vi "Multistation Example.vi"() -> ()   [LabVIEW 2019]
uses:
  Test Bench Tools.lvlib
panel:
  in  "Launch Test 2":bool
  out "Result_Station2":T1(array[cluster])
  out "Result_Station1":T1(array[cluster])
  in  "Launch Test":bool
  in  "Stop":bool
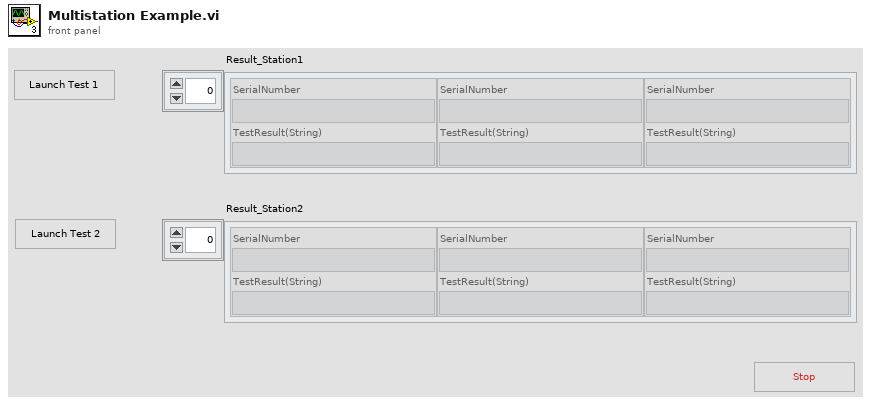
[diagram p1: front panel]
types:
  T1 = cluster{"SerialNumber":string, "TestResult(String)":string}[]
  T2 = enum16{"Station 1", "Station 2", "Station 3", "Station 4"}
  T3 = cluster{"new reference":refnum<k24>, "Array":refnum<k27>[], "Mgessage":refnum<user-event>}
  T4 = enum32{"Invalid", "Standard", "Closed", "Hidden", "Minimized", "Maximized"}
  T5 = enum32{"invalid app kind", "Development System", "Run Time System", "Student Edition", "Embedded LabVIEW", "Evaluation", "Custom"}
  T6 = cluster{"Core":cluster{"Current VI Reference":refnum<vi>, "Close Panel on Exit?":bool}, "Your Boolean data":bool, "Your string data":string, "hWnd":u32}
  T7 = cluster{"Current VI Reference":refnum<vi>, "Close Panel on Exit?":bool}
  T8 = enum16{"None", "Top", "Bottom", "Left", "Right", "Left-Top", "Left-Bottom", "Right-Top", "Right-Bottom"}[]
  T9 = cluster{"SerialNumber":string, "TestResult(String)":string}
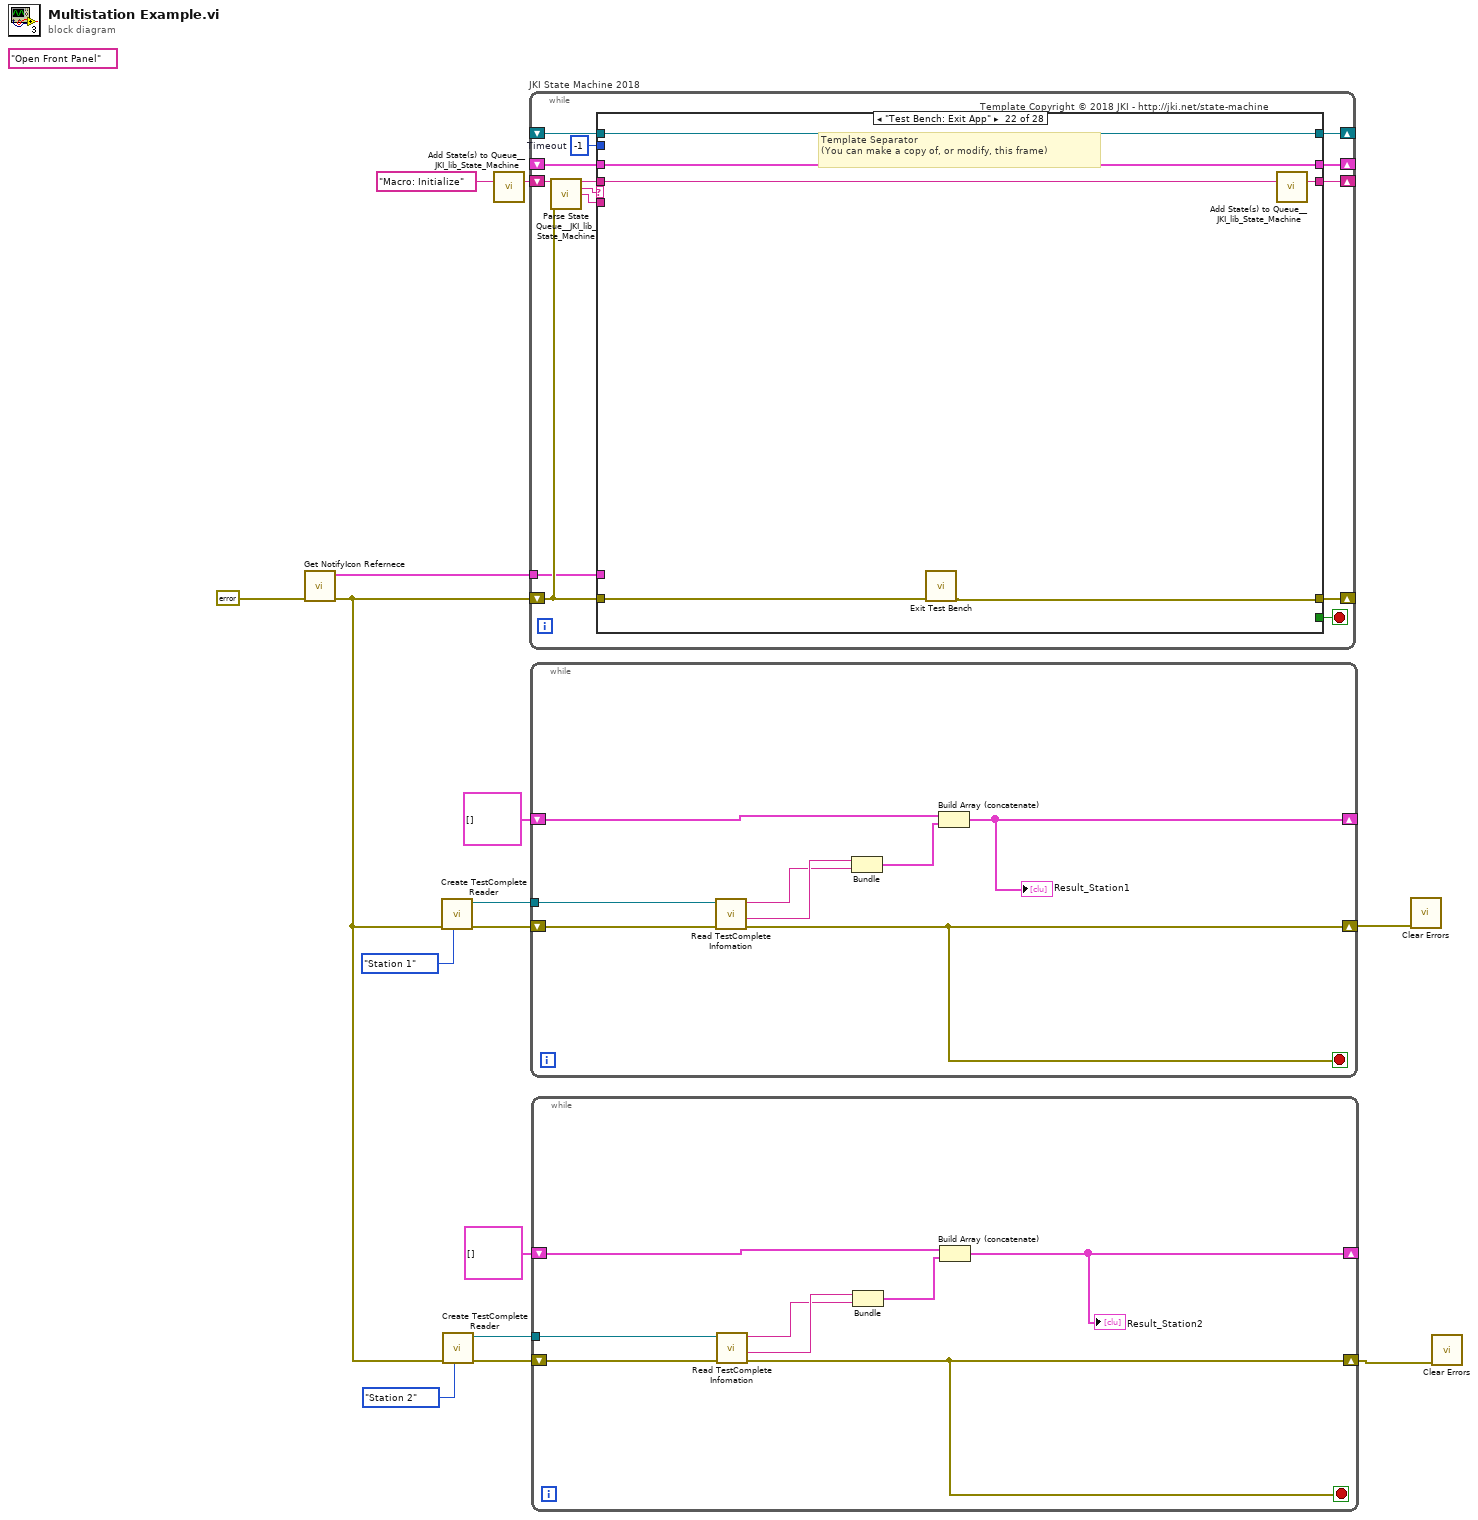
[diagram p0: block diagram]
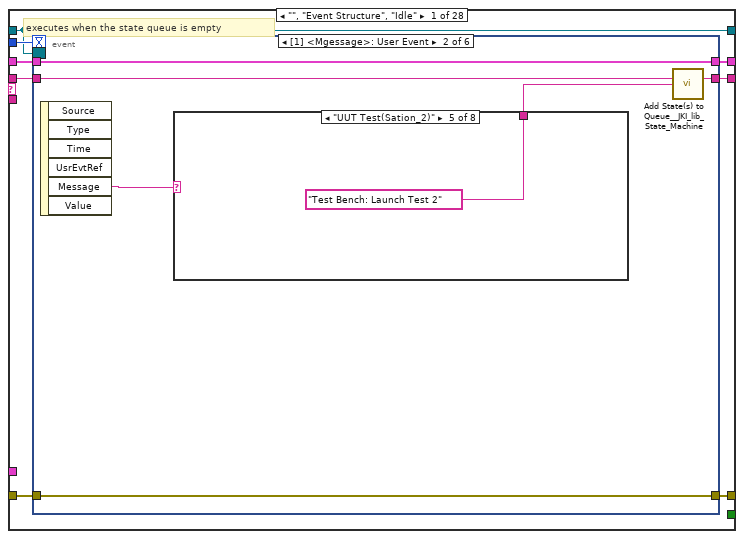
[diagram p2: hidden frame]
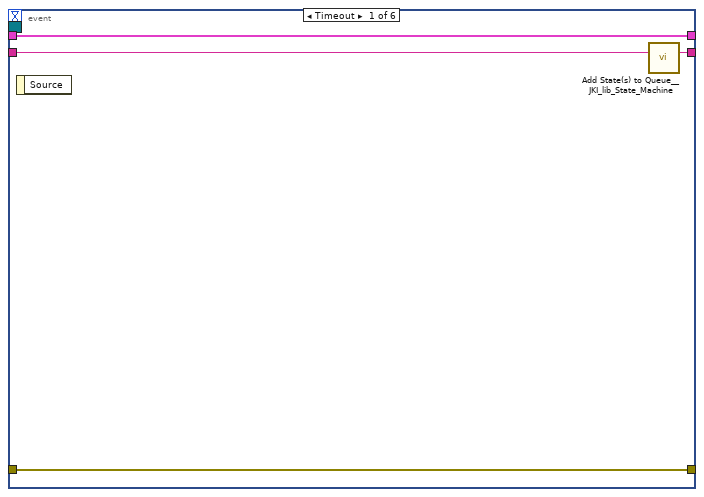
[diagram p3: hidden frame]
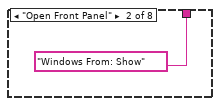
[diagram p5: hidden frame]
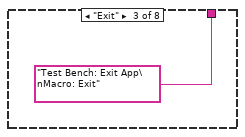
[diagram p6: hidden frame]
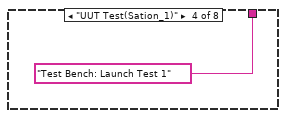
[diagram p7: hidden frame]
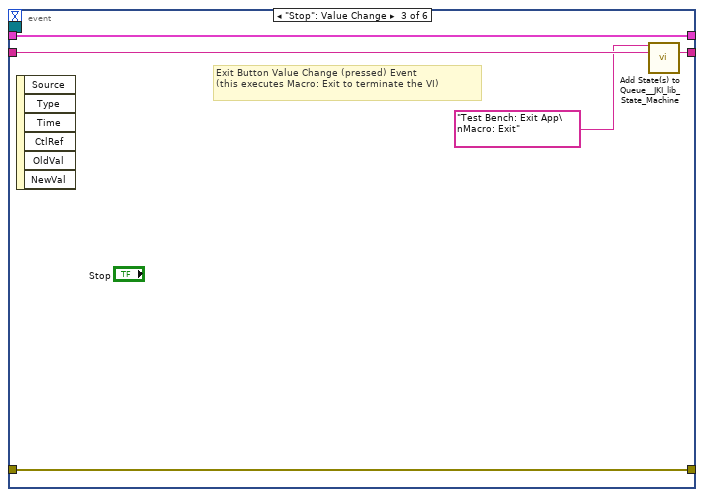
[diagram p11: hidden frame]
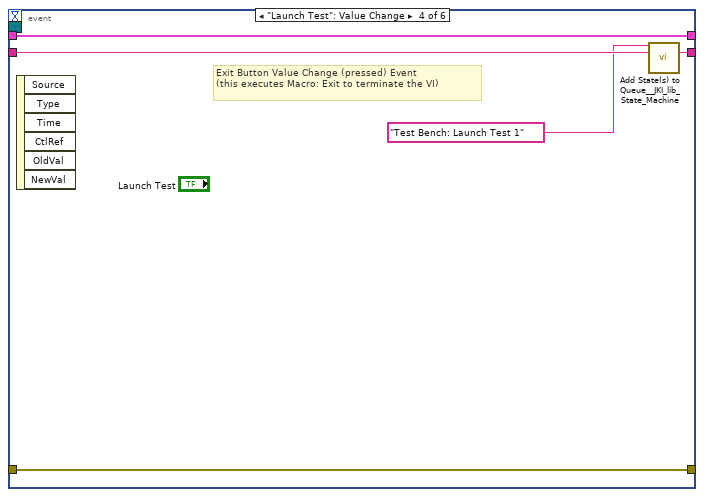
[diagram p12: hidden frame]
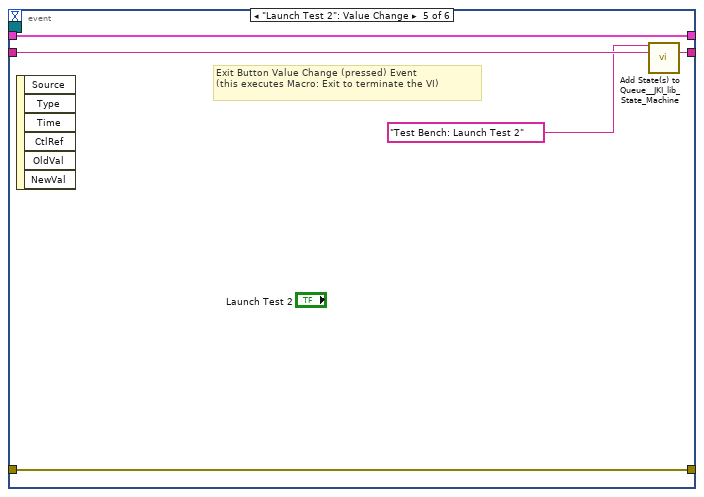
[diagram p13: hidden frame]
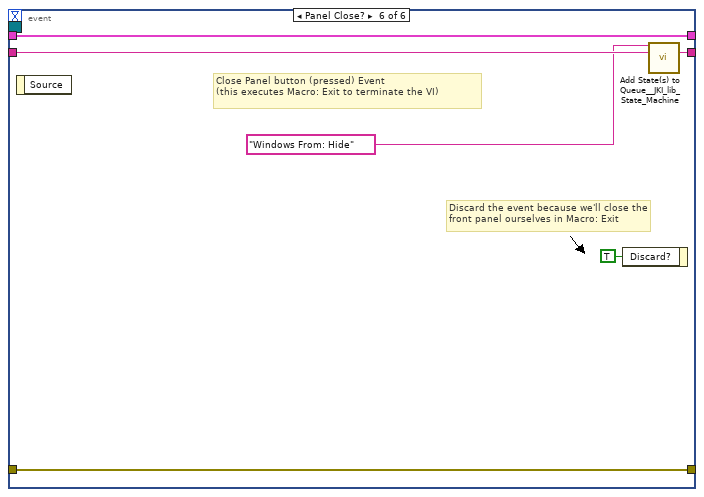
[diagram p14: hidden frame]
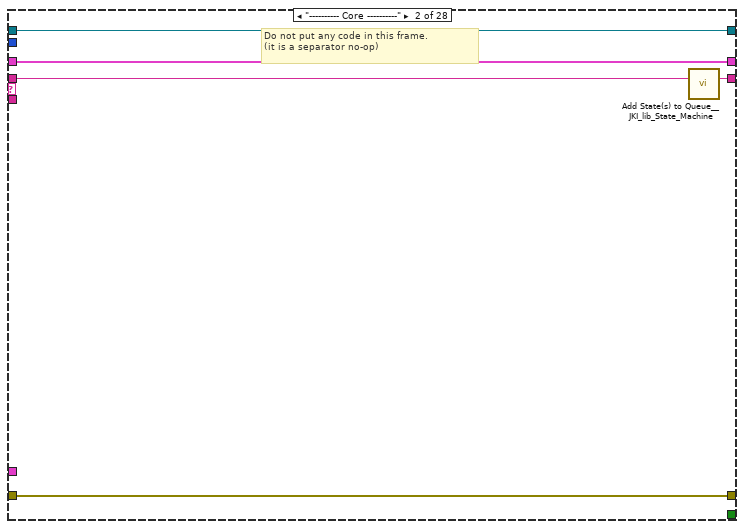
[diagram p15: hidden frame]
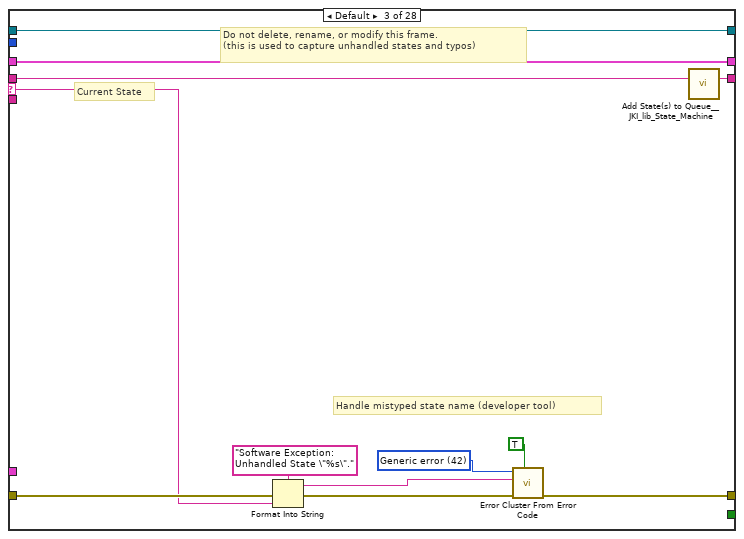
[diagram p16: hidden frame]
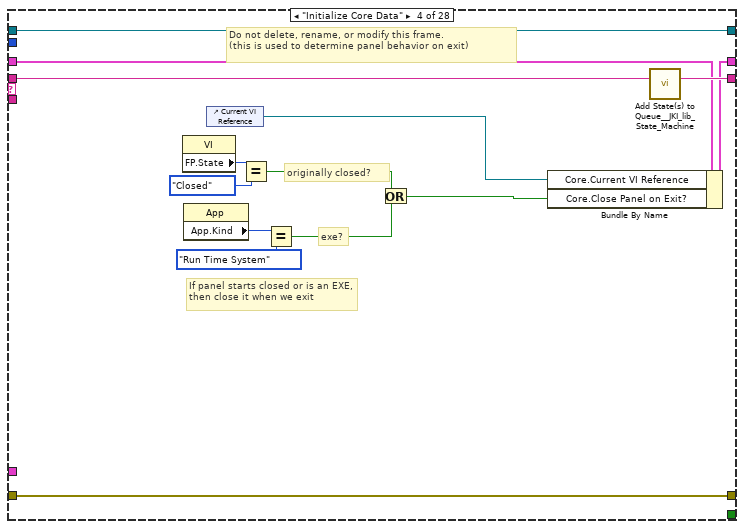
[diagram p17: hidden frame]
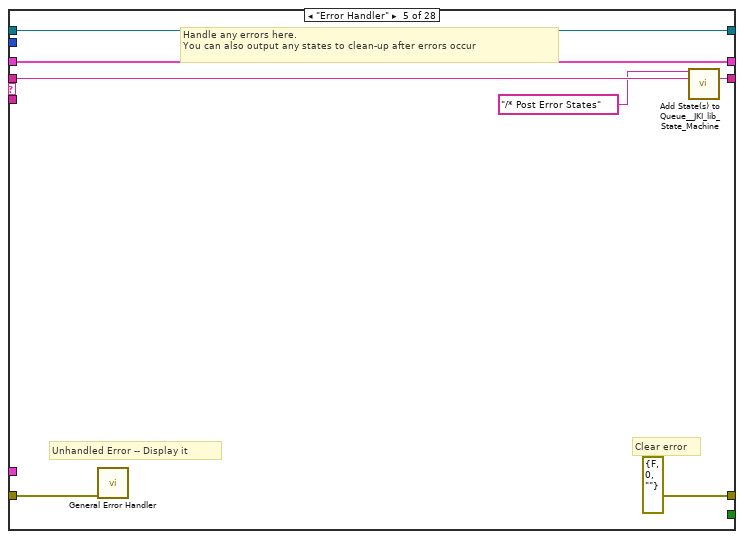
[diagram p18: hidden frame]
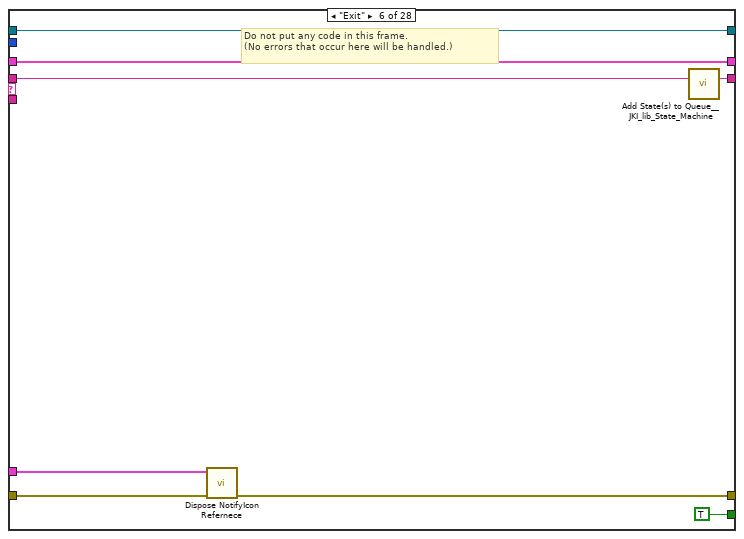
[diagram p19: hidden frame]
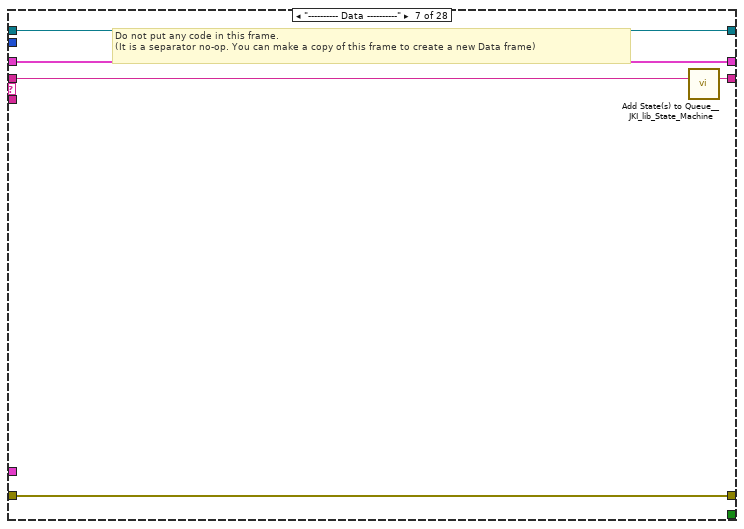
[diagram p20: hidden frame]
diagram:
  (unwired) "Open Front Panel" ("text")
  n1 = call "Get NotifyIcon Refernece.vi"("error in (no error)"=errorcluster {"status"=FALSE, "code"=0, "source"=""} ("error out")) -> ("error out"=w3:errorcluster, "reference out"=w9:T3)  [unwired: 9 in]
  n2 = call "Create TestComplete Reader.vi"("Station"=T2."Station 1", "error in (no error)"=w3) -> ("error out"=w13:errorcluster, "reader endpoint"=w11:refnum<k21>)  [unwired: 8 in]
  n3 = call "Create TestComplete Reader.vi"("Station"=T2."Station 2", "error in (no error)"=w3) -> ("error out"=w4:errorcluster, "reader endpoint"=w6:refnum<k21>)  [unwired: 8 in]
  n4 = call <vilib>:"Add State(s) to Queue__JKI_lib_State_Machine.vi"("State(s) in (\"\")"="Macro: Initialize") -> ("States Out"=w15:string)  [unwired: 14 in]
  n5 = while "JKI State Machine 2018" {
    shift-right: [w22] -> _
    shift-left: _ -> [w21]
    shift-right: [w25] -> _
    shift-left: w3 -> [w19]
    shift-right: [w24] -> _
    shift-left: w15 -> [w26]
    shift-right: [w18] -> _
    shift-left: _ -> [w17]
    tunnel: w9 -> [w16]
    stop <- w23 stop-if-true
    w20 = -1  # Timeout
    # "Template Copyright © 2018 JKI - http://jki.net/state-machine"
    n6 = call <vilib>:"Parse State Queue__JKI_lib_State_Machine.vi"("State Queue"=w26, "Error In (no error)"=w19) -> ("Remaining States"=w28:string, "Current State"=w29:string, "Arguments"=w27:string)  [unwired: 11 in]
    n7 = case shown="\"Test Bench: Exit App\"" w29 {
      selector: w29 -> [_ _ w79 _ _ _ _ _ _ _ _ _ _ _ _ _ _ _ _ _ _ _ _ _ _ _ _ _]
      tunnel: w28 -> [w37 w77 w83 w103 w110 w118 w123 w132 w139 w144 w152 w158 w163 w168 w175 w187 w257 w263 w274 w279 w286 w292 w300 w308 w313 w327 w344 w353]
      tunnel: w27 -> [_ _ _ _ _ _ _ _ _ _ _ _ _ _ w170 w181 _ _ _ _ _ _ _ _ _ _ _ _]
      tunnel: w21 -> [w35 w74 w81 w96 w107 w116 w120 _ w134 w141 w150 w156 w160 w166 w173 w183 w254 w260 w271 w276 w284 w290 w298 w306 w310 w323 w341 w347]
      tunnel: [w34 w75 w85 w100 errorcluster {"status"=FALSE, "code"=0, "source"=""} ("error out") w111 w121 w129 w135 w142 w148 w153 w161 w165 w171 w184 w255 w261 w272 w277 w282 w287 w293 w302 w309 w319 w329 w349] -> w25
      tunnel: w19 -> [w33 w75 w84 w100 w106 w112 w121 w129 w136 w142 w147 w154 w161 w165 w172 w185 w255 w261 w272 w277 w283 w289 w295 w303 w309 w324 w335 w350]
      tunnel: [w36 w76 w82 w102 w109 w117 w122 w131 w138 w143 w151 w157 w162 w167 w174 w186 w256 w262 w273 w278 w285 w291 w299 w307 w312 w326 w343 w352] -> w24
      tunnel: [_ _ _ _ _ TRUE _ _ _ _ _ _ _ _ _ _ _ _ _ _ _ _ _ _ _ _ _ _] -> w23
      tunnel: [w32 w74 w81 w101 w107 w116 w120 w130 w134 w141 w150 w156 w160 w166 w173 w183 w254 w260 w271 w276 w284 w290 w298 w306 w310 w323 w341 w345] -> w22
      tunnel: w20 -> [w31 _ _ _ _ _ _ _ _ _ _ _ _ _ _ _ _ _ _ _ _ _ _ _ _ _ _ _]
      tunnel: [w30 w73 w78 w90 w104 w114 w119 w125 w133 w140 w149 w155 w159 w164 w169 w180 w253 w258 w264 w275 w281 w288 w296 w304 w311 w325 w342 w351] -> w18
      tunnel: w17 -> [w30 w73 w78 w90 w104 w114 w119 w125 w133 w140 _ w155 w159 w164 w169 w180 w253 w258 w264 w275 w281 w288 w296 w304 w311 w325 w342 w351]
      tunnel: w16 -> [_ _ _ _ _ w113 _ _ _ _ w146 _ _ _ _ _ _ _ _ _ _ _ _ _ _ _ _ _]
      frame "", "Event Structure", "Idle" {
        # "executes when the state queue is empty"
        n8 = event shown="[1] <Mgessage>: User Event" {
          selector: w30 -> [_ _ _ _ _ _]
          dyn-events: _ -> [_ _ _ _ _ _]
          timeout: w31 -> [_ _ _ _ _ _]
          tunnel: w37 -> [w41 w47 w56 w61 w66 w72]
          tunnel: [w40 w46 w55 w60 w65 w71] -> w36
          tunnel: w35 -> [w38 w44 w53 w58 w63 w69]
          tunnel: [w39 w45 w54 w59 w64 w70] -> w34
          tunnel: w33 -> [w39 w45 w54 w59 w64 w70]
          tunnel: [w38 w44 w53 w58 w63 w69] -> w32
          event Timeout {
            n9 = event-data() -> ()  [unwired: 1 in, 1 out]
            n10 = call <vilib>:"Add State(s) to Queue__JKI_lib_State_Machine.vi"("State(s) in (\"\")"=w41) -> ("States Out"=w40:string)  [unwired: 14 in]
          }
          event User Event {
            n11 = event-data() -> ("Message"=w43:string)  [unwired: 1 in, 5 out]
            n12 = case shown="\"UUT Test(Sation_2)\"" w43 {
              tunnel: [_ "Windows From: Show" "Test Bench: Exit App\nMacro: Exit" "Test Bench: Launch Test 1" "Test Bench: Launch Test 2" _ _ _] -> w42
              frame "Idle", Default {
              }
              frame "Open Front Panel" {
              }
              frame "Exit" {
              }
              frame "UUT Test(Sation_1)" {
              }
              frame "UUT Test(Sation_2)" {
              }
              frame "UUT Test(Sation_3)" {
              }
              frame "UUT Test(Sation_4)" {
              }
              frame "Select Sequence(Sation_1)" {
              }
            }
            n13 = call <vilib>:"Add State(s) to Queue__JKI_lib_State_Machine.vi"("State(s) in (\"\")"=w47, "State(s) at Back (\"\")"=w42) -> ("States Out"=w46:string)  [unwired: 13 in]
          }
          event "Stop": Value Change {
            # "Exit Button Value Change (pressed) Event\n(this executes Macro: Exit to terminate the VI)"
            n14 = event-data() -> ()  [unwired: 1 in, 6 out]
            n15 = call <vilib>:"Add State(s) to Queue__JKI_lib_State_Machine.vi"("State(s) in Front (\"\")"="Test Bench: Exit App\nMacro: Exit", "State(s) in (\"\")"=w56) -> ("States Out"=w55:string)  [unwired: 13 in]
          }
          event "Launch Test": Value Change {
            # "Exit Button Value Change (pressed) Event\n(this executes Macro: Exit to terminate the VI)"
            n16 = event-data() -> ()  [unwired: 1 in, 6 out]
            n17 = call <vilib>:"Add State(s) to Queue__JKI_lib_State_Machine.vi"("State(s) in Front (\"\")"="Test Bench: Launch Test 1", "State(s) in (\"\")"=w61) -> ("States Out"=w60:string)  [unwired: 13 in]
          }
          event "Launch Test 2": Value Change {
            # "Exit Button Value Change (pressed) Event\n(this executes Macro: Exit to terminate the VI)"
            n18 = event-data() -> ()  [unwired: 1 in, 6 out]
            n19 = call <vilib>:"Add State(s) to Queue__JKI_lib_State_Machine.vi"("State(s) in Front (\"\")"="Test Bench: Launch Test 2", "State(s) in (\"\")"=w66) -> ("States Out"=w65:string)  [unwired: 13 in]
          }
          event Panel Close? {
            # "Discard the event because we'll close the front panel ourselves in Macro: Exit"
            # "Close Panel button (pressed) Event\n(this executes Macro: Exit to terminate the VI)"
            n20 = event-data() -> ()  [unwired: 1 in, 1 out]
            n21 = event-data("Discard?"=TRUE) -> ()  [unwired: 1 in, 1 out]
            n22 = call <vilib>:"Add State(s) to Queue__JKI_lib_State_Machine.vi"("State(s) in Front (\"\")"="Windows From: Hide", "State(s) in (\"\")"=w72) -> ("States Out"=w71:string)  [unwired: 13 in]
          }
        }
      }
      frame "---------- Core ----------" {
        # "Do not put any code in this frame.\n(it is a separator no-op)"
        n23 = call <vilib>:"Add State(s) to Queue__JKI_lib_State_Machine.vi"("State(s) in (\"\")"=w77) -> ("States Out"=w76:string)  [unwired: 14 in]
      }
      frame Default {
        w88 = 42 items=["No error", "Argument error", "Memory is full", "Out of zone", "End of file", "File already open", "Generic file I/O error", "File not found", "File permission error", "Disk is full", "Duplicate path", "Too many files open", "System feature not enabled", "Resource file not found", "Cannot add resource", "Resource not found", "Image not found", "Image memory error", "Pen does not exist", "Config type invalid", "Config token not found", "Config parse error", "Config memory error", "Bad external code format", "Bad external code offset", "External code not present", "Null window", "Destroy window error", "Null menu", "Print aborted", "Bad print record", "Print driver error", "Windows error during printing", "Memory error during printing", "Print dialog error", "Generic print error", "Invalid device refnum", "Device not found", "Device parameter error", "Device unit error", "Cannot open device", "Device call aborted", "Generic error", "Cancelled by user", "Object ID too low", "Object ID too high", "Object not in heap", "Unknown heap", "Unknown object (invalid DefProc)", "Unknown object (DefProc not in table)", "Message out of range", "Invalid (null) method", "Unknown message", "Manager call not supported", "Bad address", "Network operation in progress", "Network operation timed out", "Connection is busy", "Network attribute not supported", "Network error", "Address in use", "System out of memory", "Connection aborted", "Connection refused", "Not connected", "Already connected", "Connection closed", "Initialization error (interapplication manager)", "Bad occurrence", "Wait on unbound occurrence handler", "Occurrence queue overflow", "Datalog type conflict", "Unused", "Unrecognized type (interapplication manager)", "Memory corrupt", "Failed to make temporary DLL", "Old CIN version", "Drag socket not found", "Failed to load drop-object", "Failed to register OLE object", "Failed to release OLE object", "Format specifier type mismatch", "Unknown format specifier", "Too few format specifiers", "Too many format specifiers", "Scan failed", "Newer CIN version", "Error converting to variant", "Runtime menu error", "Password tampered", "Variant attribute not found", "Incompatible variant data type", "Event data is not available", "Event Store is not present", "Occurrence is not found", "Event Queue is not created", "Event info is not available", "Refnum passed is NULL", "Error retrieving Class GUID", "Error retrieving CoClass GUID", "Error retrieving TypeLib GUID.", "Bad built application magic bytes.", "Specific driver is different from the specific driver associated with the Logical Name.", "There is no session opened to the class driver.", "Max Error", "MAX - Error with config objects", "MAX - Error loading configuration", "MAX - Group not supported"]
        # "Current State"
        # "Do not delete, rename, or modify this frame.\n(this is used to capture unhandled states and typos)"
        # "Handle mistyped state name (developer tool)"
        n24 = Format Into String(format string="Software Exception: Unhandled State \"%s\"." ("message"), error in=w84, w79) -> (resulting string=w87:string, error out=w86:errorcluster)  [unwired: 1 in]
        n25 = call <vilib>:"Error Cluster From Error Code.vi"("show call chain? (False)"=TRUE, "error in (no error)"=w86, "error message (\"\")"=w87, "error code (0)"=w88) -> ("error out"=w85:errorcluster)  [unwired: 5 in]
        n26 = call <vilib>:"Add State(s) to Queue__JKI_lib_State_Machine.vi"("State(s) in (\"\")"=w83) -> ("States Out"=w82:string)  [unwired: 14 in]
      }
      frame "Initialize Core Data" {
        # "Do not delete, rename, or modify this frame.\n(this is used to determine panel behavior on exit)"
        # "originally closed?"
        # "exe?"
        # "If panel starts closed or is an EXE, then close it when we exit"
        n27 = property class="VI"() -> ("FP.State"=w93:T4)  [unwired: 2 in, 2 out]
        n28 = property class="App"() -> ("App.Kind"=w99:T5)  [unwired: 2 in, 2 out]
        n29 = control-ref of="Current VI Reference"() -> (w94:refnum<vi>)
        n30 = Equal?(x=w93, y=T4."Closed" ("Front Panel Window:State")) -> (x = y?=w91:bool)
        n31 = Equal?(x=w99, y=T5."Run Time System" ("Application:Kind")) -> (x = y?=w97:bool)
        n32 = Or(x=w91, y=w97) -> (x .or. y?=w95:bool)
        n33 = Bundle By Name(cluster=w96, "Core.Current VI Reference"=w94, "Core.Close Panel on Exit?"=w95) -> (w101:T6)
        n34 = call <vilib>:"Add State(s) to Queue__JKI_lib_State_Machine.vi"("State(s) in (\"\")"=w103) -> ("States Out"=w102:string)  [unwired: 14 in]
      }
      frame "Error Handler" {
        # "Unhandled Error -- Display it"
        # "Handle any errors here.\nYou can also output any states to clean-up after errors occur"
        # "Clear error"
        n35 = call <vilib>:"General Error Handler.vi"("error in (no error)"=w106) -> ()  [unwired: 10 in, 5 out]
        n36 = call <vilib>:"Add State(s) to Queue__JKI_lib_State_Machine.vi"("State(s) in Front (\"\")"="/* Post Error States", "State(s) in (\"\")"=w110) -> ("States Out"=w109:string)  [unwired: 13 in]
      }
      frame "Exit" {
        # "Do not put any code in this frame.\n(No errors that occur here will be handled.)"
        n37 = call "Dispose NotifyIcon Refernece.vi"("error in (no error)"=w112, "reference"=w113) -> ("error out"=w111:errorcluster)  [unwired: 9 in]
        n38 = call <vilib>:"Add State(s) to Queue__JKI_lib_State_Machine.vi"("State(s) in (\"\")"=w118) -> ("States Out"=w117:string)  [unwired: 14 in]
      }
      frame "---------- Data ----------" {
        # "Do not put any code in this frame.\n(It is a separator no-op. You can make a copy of this frame to create a new Data frame)"
        n39 = call <vilib>:"Add State(s) to Queue__JKI_lib_State_Machine.vi"("State(s) in (\"\")"=w123) -> ("States Out"=w122:string)  [unwired: 14 in]
      }
      frame "Data: Initialize" {
        w124 = u32 0  # hWnd
        w126 = T7 {"Current VI Reference"=refnum, "Close Panel on Exit?"=FALSE}  # Core
        w128 = TRUE  # Your Boolean data
        w127 = ""  # Your string data
        # "do not delete - used by framework"
        # "Add new data here."
        # "Data names and types of shift register data are defined by this bundle."
        # "Initialize the shift-register data, here.\n(data names are defined by what you wire into the bundle function)"
        n40 = Bundle("Core"=w126, "Your Boolean data"=w128, "Your string data"=w127, "hWnd"=w124) -> (w130:T6)  [unwired: 1 in]
        n41 = call <vilib>:"Add State(s) to Queue__JKI_lib_State_Machine.vi"("State(s) in (\"\")"=w132) -> ("States Out"=w131:string)  [unwired: 14 in]
      }
      frame "Data: Cleanup" {
        # "Cleanup any data and references, here.\n(this is called automatically, by the Macro: Exit)"
        n42 = Unbundle By Name(w134) -> ("Core.Current VI Reference"=w137:refnum<vi>)
        n43 = Close Reference(reference=w137, error in (no error)=w136) -> (error out=w135:errorcluster)
        n44 = call <vilib>:"Add State(s) to Queue__JKI_lib_State_Machine.vi"("State(s) in (\"\")"=w139) -> ("States Out"=w138:string)  [unwired: 14 in]
      }
      frame "---------- Events ----------" {
        # "Do not put any code in this frame.\n(It is a separator no-op. You can make a copy of this frame to create a new UI frame)"
        n45 = call <vilib>:"Add State(s) to Queue__JKI_lib_State_Machine.vi"("State(s) in (\"\")"=w144) -> ("States Out"=w143:string)  [unwired: 14 in]
      }
      frame "Events: Register" {
        # "Do not put any code in this frame.\n(It is a separator no-op. You can make a copy of this frame to create a new UI frame)"
        n46 = Unbundle By Name(w146) -> ("Mgessage"=w145:refnum<user-event>)
        n47 = register-events(error in=w147, w145) -> (reference out=w149:refnum<event-registration>, error out=w148:errorcluster)  [unwired: 1 in]
        n48 = call <vilib>:"Add State(s) to Queue__JKI_lib_State_Machine.vi"("State(s) in (\"\")"=w152) -> ("States Out"=w151:string)  [unwired: 14 in]
      }
      frame "Events: Unregister" {
        # "Do not put any code in this frame.\n(It is a separator no-op. You can make a copy of this frame to create a new UI frame)"
        n49 = Unregister For Events(event registration refnum=w155, error in=w154) -> (error out=w153:errorcluster)
        n50 = call <vilib>:"Add State(s) to Queue__JKI_lib_State_Machine.vi"("State(s) in (\"\")"=w158) -> ("States Out"=w157:string)  [unwired: 14 in]
      }
      frame "---------- UI ----------" {
        # "Do not put any code in this frame.\n(It is a separator no-op. You can make a copy of this frame to create a new UI frame)"
        n51 = call <vilib>:"Add State(s) to Queue__JKI_lib_State_Machine.vi"("State(s) in (\"\")"=w163) -> ("States Out"=w162:string)  [unwired: 14 in]
      }
      frame "UI: Initialize" {
        # "Initialize the User Interface, here.\n(this is called automatically, by the Macro: Init)"
        n52 = call <vilib>:"Add State(s) to Queue__JKI_lib_State_Machine.vi"("State(s) in (\"\")"=w168) -> ("States Out"=w167:string)  [unwired: 14 in]
      }
      frame "UI: Cursor Set" {
        # "Argument"
        # "Set and Unset Cursor Busy.\n(Usage: \"UI: Cursor Set >> Busy|Idle\")"
        n53 = case shown="\"Idle\", Default" w170 {
          tunnel: w172 -> [w177 w179]
          tunnel: [w176 w178] -> w171
          frame "Idle", Default {
            n54 = call <vilib>:"Unset Busy.vi"("error in (no error)"=w177) -> ("error out"=w176:errorcluster)  [unwired: 10 in]
          }
          frame "Busy" {
            n55 = call <vilib>:"Set Busy.vi"("error in (no error)"=w179) -> ("error out"=w178:errorcluster)  [unwired: 9 in, 1 out]
          }
        }
        n56 = call <vilib>:"Add State(s) to Queue__JKI_lib_State_Machine.vi"("State(s) in (\"\")"=w175) -> ("States Out"=w174:string)  [unwired: 14 in]
      }
      frame "UI: Front Panel State" {
        # "Argument"
        # "Set Front Panel Open or Closed\n(Usage: \"UI: Front Panel State >> Open|Close\")"
        n57 = Unbundle By Name(w183) -> ("Core.Current VI Reference"=w182:refnum<vi>)
        n58 = case shown="\"Minimize\", \"Minimized\"" w181 {
          tunnel: w185 -> [w193 w208 w219 w232 w245]
          tunnel: [w195 w209 w221 w234 w247] -> w184
          tunnel: w182 -> [w194 w206 w220 w233 w246]
          frame "Open", "Standard", Default {
            w188 = T4."Standard" ("State")
            n59 = property class="VI"(reference=w194, error in=w193) -> (reference out=w191:refnum<vi>, error out=w192:errorcluster, "FP.State"=w190:T4)
            n60 = Not Equal?(x=w190, y=w188) -> (x != y?=w189:bool)
            n61 = case shown="True" w189 {
              tunnel: [w199 w201] -> w195
              tunnel: w192 -> [w198 w201]
              tunnel: w191 -> [w197 _]
              tunnel: w188 -> [w196 _]
              frame True {
                n62 = invoke class="VI" method="FP.Open"(reference=w197, error in=w198, "Activate"=TRUE, "State"=w196) -> (error out=w199:errorcluster)  [unwired: 1 in, 4 out]
              }
              frame False {
              }
            }
          }
          frame "Close", "Closed" {
            n63 = property class="VI"(reference=w206, error in=w208) -> (reference out=w205:refnum<vi>, error out=w207:errorcluster, "FP.State"=w203:T4)
            n64 = Not Equal?(x=w203, y=T4."Closed" ("Front Panel Window:State")) -> (x != y?=w202:bool)
            n65 = case shown="True" w202 {
              tunnel: [w210 w213] -> w209
              tunnel: w207 -> [w210 w212]
              tunnel: w205 -> [_ w211]
              frame False {
              }
              frame True {
                n66 = invoke class="VI" method="FP.Close"(reference=w211, error in=w212) -> (error out=w213:errorcluster)  [unwired: 1 in, 2 out]
              }
            }
          }
          frame "Hidden", "Hide" {
            w214 = T4."Hidden" ("State")
            n67 = property class="VI"(reference=w220, error in=w219) -> (reference out=w217:refnum<vi>, error out=w218:errorcluster, "FP.State"=w216:T4)
            n68 = Not Equal?(x=w216, y=w214) -> (x != y?=w215:bool)
            n69 = case shown="True" w215 {
              tunnel: [w225 w226] -> w221
              tunnel: w218 -> [w224 w226]
              tunnel: w217 -> [w223 _]
              tunnel: w214 -> [w222 _]
              frame True {
                n70 = invoke class="VI" method="FP.Open"(reference=w223, error in=w224, "State"=w222) -> (error out=w225:errorcluster)  [unwired: 2 in, 4 out]
              }
              frame False {
              }
            }
          }
          frame "Minimize", "Minimized" {
            w227 = T4."Minimized" ("State")
            n71 = property class="VI"(reference=w233, error in=w232) -> (reference out=w230:refnum<vi>, error out=w231:errorcluster, "FP.State"=w229:T4)
            n72 = Not Equal?(x=w229, y=w227) -> (x != y?=w228:bool)
            n73 = case shown="True" w228 {
              tunnel: [w238 w239] -> w234
              tunnel: w231 -> [w237 w239]
              tunnel: w230 -> [w236 _]
              tunnel: w227 -> [w235 _]
              frame True {
                n74 = invoke class="VI" method="FP.Open"(reference=w236, error in=w237, "State"=w235) -> (error out=w238:errorcluster)  [unwired: 2 in, 4 out]
              }
              frame False {
              }
            }
          }
          frame "Maximize", "Maximized" {
            w240 = T4."Maximized" ("State")
            n75 = property class="VI"(reference=w246, error in=w245) -> (reference out=w243:refnum<vi>, error out=w244:errorcluster, "FP.State"=w242:T4)
            n76 = Not Equal?(x=w242, y=w240) -> (x != y?=w241:bool)
            n77 = case shown="True" w241 {
              tunnel: [w251 w252] -> w247
              tunnel: w244 -> [w250 w252]
              tunnel: w243 -> [w249 _]
              tunnel: w240 -> [w248 _]
              frame True {
                n78 = invoke class="VI" method="FP.Open"(reference=w249, error in=w250, "State"=w248) -> (error out=w251:errorcluster)  [unwired: 2 in, 4 out]
              }
              frame False {
              }
            }
          }
        }
        n79 = call <vilib>:"Add State(s) to Queue__JKI_lib_State_Machine.vi"("State(s) in (\"\")"=w187) -> ("States Out"=w186:string)  [unwired: 14 in]
      }
      frame "---------- Macro ----------" {
        # "Do not put any code in this frame.\n(It is a separator no-op. You can make a copy of this frame to create a new Macro frame)"
        n80 = call <vilib>:"Add State(s) to Queue__JKI_lib_State_Machine.vi"("State(s) in (\"\")"=w257) -> ("States Out"=w256:string)  [unwired: 14 in]
      }
      frame "Macro: Initialize" {
        # "Initialization Macro\n(This is called once, when the VI starts)"
        n81 = call <vilib>:"Add State(s) to Queue__JKI_lib_State_Machine.vi"("State(s) in Front (\"\")"="Data: Initialize\nInitialize Core Data\nEvents: Register\nUI: Initialize\nUI: Front Panel State >> Open\nTest Bench: Launch Test Bench\nWindows From: Find Windows\nWindows From: Hide", "State(s) in (\"\")"=w263) -> ("States Out"=w262:string)  [unwired: 13 in]
      }
      frame "Macro: Exit" {
        # "Exit Macro\n(This is called once, when the VI exits)"
        n82 = Unbundle By Name(w271) -> ("Core.Close Panel on Exit?"=w270:bool)
        n83 = Select(t="UI: Front Panel State >> Close", s=w270, f="") -> (s? t:f=w267:string)
        n84 = call <vilib>:"Add State(s) to Queue__JKI_lib_State_Machine.vi"("State(s) in (\"\")"=w267, "State(s) at Back (\"\")"="Data: Cleanup\nEvents: Unregister\nExit") -> ("States Out"=w265:string)  [unwired: 13 in]
        n85 = call <vilib>:"Add State(s) to Queue__JKI_lib_State_Machine.vi"("State(s) in Front (\"\")"=w265, "State(s) in (\"\")"=w274) -> ("States Out"=w273:string)  [unwired: 13 in]
      }
      frame "---------- Test Bench ----------" {
        # "Template Separator\n(You can make a copy of, or modify, this frame)"
        n86 = call <vilib>:"Add State(s) to Queue__JKI_lib_State_Machine.vi"("State(s) in (\"\")"=w279) -> ("States Out"=w278:string)  [unwired: 14 in]
      }
      frame "Test Bench: Launch Test Bench" {
        w280 = T8 [enum."Top", enum."Bottom"] items=["None", "Top", "Bottom", "Left", "Right", "Left-Top", "Left-Bottom", "Right-Top", "Right-Bottom"] ("Position")
        # "Template Separator\n(You can make a copy of, or modify, this frame)"
        n87 = call "Launch Test Bench.vi"("Position"=w280, "error in (no error)"=w283) -> ("error out"=w282:errorcluster)  [unwired: 9 in]
        n88 = call <vilib>:"Add State(s) to Queue__JKI_lib_State_Machine.vi"("State(s) in (\"\")"=w286) -> ("States Out"=w285:string)  [unwired: 14 in]
      }
      frame "Test Bench: Exit App" {
        # "Template Separator\n(You can make a copy of, or modify, this frame)"
        n89 = call "Exit Test Bench.vi"("error in (no error)"=w289) -> ("error out"=w287:errorcluster)  [unwired: 10 in]
        n90 = call <vilib>:"Add State(s) to Queue__JKI_lib_State_Machine.vi"("State(s) in (\"\")"=w292) -> ("States Out"=w291:string)  [unwired: 14 in]
      }
      frame "Test Bench: Launch Test 1" {
        # "Template Separator\n(You can make a copy of, or modify, this frame)"
        n91 = call "Launch Test.vi"("Station"=T2."Station 1", "error in (no error)"=w295) -> ("error out"=w293:errorcluster)  [unwired: 9 in]
        n92 = property on="Result_Station1" class="Arr (strict)"("Value"=T1 [] ("Array")) -> ()  [unwired: 2 in, 2 out]
        n93 = call <vilib>:"Add State(s) to Queue__JKI_lib_State_Machine.vi"("State(s) in (\"\")"=w300) -> ("States Out"=w299:string)  [unwired: 14 in]
      }
      frame "Test Bench: Launch Test 2" {
        # "Template Separator\n(You can make a copy of, or modify, this frame)"
        n94 = call "Launch Test.vi"("Station"=T2."Station 2", "error in (no error)"=w303) -> ("error out"=w302:errorcluster)  [unwired: 9 in]
        n95 = property on="Result_Station2" class="Arr (strict)"("Value"=T1 [] ("Array")) -> ()  [unwired: 2 in, 2 out]
        n96 = call <vilib>:"Add State(s) to Queue__JKI_lib_State_Machine.vi"("State(s) in (\"\")"=w308) -> ("States Out"=w307:string)  [unwired: 14 in]
      }
      frame "---------- Windows From ----------" {
        # "Template Separator\n(You can make a copy of, or modify, this frame)"
        n97 = call <vilib>:"Add State(s) to Queue__JKI_lib_State_Machine.vi"("State(s) in (\"\")"=w313) -> ("States Out"=w312:string)  [unwired: 14 in]
      }
      frame "Windows From: Show" {
        w315 = u32 2 items=["SWP_ASYNCWINDOWPOS"=16384, "SWP_DEFERERASE"=8192, "SWP_DRAWFRAME"=32, "SWP_HIDEWINDOW"=128, "SWP_NOACTIVATE"=16, "SWP_NOCOPYBITS"=256, "SWP_NOMOVE"=2, "SWP_NOOWNERZORDER"=512, "SWP_NOREDRAW"=8, "SWP_NOSENDCHANGING"=1024, "SWP_NOSIZE"=1, "SWP_NOZORDER"=4, "SWP_SHOWWINDOW"=64] ("uFlags")
        w316 = u32 1 items=["SWP_ASYNCWINDOWPOS"=16384, "SWP_DEFERERASE"=8192, "SWP_DRAWFRAME"=32, "SWP_HIDEWINDOW"=128, "SWP_NOACTIVATE"=16, "SWP_NOCOPYBITS"=256, "SWP_NOMOVE"=2, "SWP_NOOWNERZORDER"=512, "SWP_NOREDRAW"=8, "SWP_NOSENDCHANGING"=1024, "SWP_NOSIZE"=1, "SWP_NOZORDER"=4, "SWP_SHOWWINDOW"=64] ("uFlags")
        # "Template Separator\n(You can make a copy of, or modify, this frame)"
        n98 = Unbundle By Name(w323) -> ("hWnd"=w322:u32)
        n99 = Or(x=w316, y=w315) -> (x .or. y?=w314:u32)
        n100 = call "Show Windows.vi"("nCmdShow"="SW_SHOWNORMAL", "error in (no error)"=w324, "hWnd"=w322) -> ("error out"=w320:errorcluster, "hWnd out"=w318:u32)  [unwired: 7 in]
        n101 = call "Set Windows Position.vi"("error in (no error)"=w320, "uFlags"=w314, "hWndInsertAfter"="-1", "hWnd"=w318) -> ("error out"=w319:errorcluster)  [unwired: 6 in, 1 out]
        n102 = call <vilib>:"Add State(s) to Queue__JKI_lib_State_Machine.vi"("State(s) in (\"\")"=w327) -> ("States Out"=w326:string)  [unwired: 14 in]
      }
      frame "Windows From: Hide" {
        w338 = u32 2 items=["SWP_ASYNCWINDOWPOS"=16384, "SWP_DEFERERASE"=8192, "SWP_DRAWFRAME"=32, "SWP_HIDEWINDOW"=128, "SWP_NOACTIVATE"=16, "SWP_NOCOPYBITS"=256, "SWP_NOMOVE"=2, "SWP_NOOWNERZORDER"=512, "SWP_NOREDRAW"=8, "SWP_NOSENDCHANGING"=1024, "SWP_NOSIZE"=1, "SWP_NOZORDER"=4, "SWP_SHOWWINDOW"=64] ("uFlags")
        w339 = u32 1 items=["SWP_ASYNCWINDOWPOS"=16384, "SWP_DEFERERASE"=8192, "SWP_DRAWFRAME"=32, "SWP_HIDEWINDOW"=128, "SWP_NOACTIVATE"=16, "SWP_NOCOPYBITS"=256, "SWP_NOMOVE"=2, "SWP_NOOWNERZORDER"=512, "SWP_NOREDRAW"=8, "SWP_NOSENDCHANGING"=1024, "SWP_NOSIZE"=1, "SWP_NOZORDER"=4, "SWP_SHOWWINDOW"=64] ("uFlags")
        # "Template Separator\n(You can make a copy of, or modify, this frame)"
        n103 = Unbundle By Name(w341) -> ("hWnd"=w336:u32)
        n104 = Or(x=w339, y=w338) -> (x .or. y?=w337:u32)
        n105 = call "Set Windows Position.vi"("error in (no error)"=w335, "uFlags"=w337, "hWndInsertAfter"="-2", "hWnd"=w336) -> ("error out"=w333:errorcluster, "hWnd out"=w334:u32)  [unwired: 6 in]
        n106 = call "Show Windows.vi"("nCmdShow"="SW_SHOWMINIMIZED", "error in (no error)"=w333, "hWnd"=w334) -> ("error out"=w331:errorcluster, "hWnd out"=w330:u32)  [unwired: 7 in]
        n107 = call "Show Windows.vi"("nCmdShow"="SW_HIDE", "error in (no error)"=w331, "hWnd"=w330) -> ("error out"=w329:errorcluster)  [unwired: 7 in, 1 out]
        n108 = call <vilib>:"Add State(s) to Queue__JKI_lib_State_Machine.vi"("State(s) in (\"\")"=w344) -> ("States Out"=w343:string)  [unwired: 14 in]
      }
      frame "Windows From: Find Windows" {
        # "Template Separator\n(You can make a copy of, or modify, this frame)"
        n109 = Unbundle By Name(w347) -> ("Core.Current VI Reference"=w348:refnum<vi>)
        n110 = call "Find Windows.vi"("error in (no error)"=w350, "VI reference"=w348) -> ("error out"=w349:errorcluster, "hWnd"=w346:u32)  [unwired: 8 in]
        n111 = Bundle By Name(cluster=w347, "hWnd"=w346) -> (w345:T6)
        n112 = call <vilib>:"Add State(s) to Queue__JKI_lib_State_Machine.vi"("State(s) in (\"\")"=w353) -> ("States Out"=w352:string)  [unwired: 14 in]
      }
    }
  }
  n113 = while {
    tunnel: w11 -> [w361]
    shift-right: [w359] -> w2
    shift-left: w13 -> [w360]
    shift-right: [w354] -> _
    shift-left: T1 [] -> [w355]
    stop <- w359 stop-if-true
    n114 = call "Read TestComplete Infomation.vi"("error in (no error)"=w360, "endpoint in"=w361) -> ("error out"=w359:errorcluster, "SerialNumber"=w358:string, "TestResult(String)"=w357:string)  [unwired: 5 in, 2 out]
    n115 = Bundle("SerialNumber"=w358, "TestResult(String)"=w357) -> (w356:T9)  [unwired: 1 in]
    n116 = Build Array (concatenate)(w355, w356) -> (w354:T1)
    "Result_Station1" <- w354
  }
  n117 = while {
    tunnel: w6 -> [w369]
    shift-right: [w367] -> w1
    shift-left: w4 -> [w368]
    shift-right: [w362] -> _
    shift-left: T1 [] -> [w363]
    stop <- w367 stop-if-true
    n118 = call "Read TestComplete Infomation.vi"("error in (no error)"=w368, "endpoint in"=w369) -> ("error out"=w367:errorcluster, "SerialNumber"=w366:string, "TestResult(String)"=w365:string)  [unwired: 5 in, 2 out]
    n119 = Bundle("SerialNumber"=w366, "TestResult(String)"=w365) -> (w364:T9)  [unwired: 1 in]
    n120 = Build Array (concatenate)(w363, w364) -> (w362:T1)
    "Result_Station2" <- w362
  }
  n121 = call <vilib>:"Clear Errors.vi"("error in (no error)"=w2) -> ()  [unwired: 5 in, 2 out]
  n122 = call <vilib>:"Clear Errors.vi"("error in (no error)"=w1) -> ()  [unwired: 5 in, 2 out]
